vi "Joint Limits.vi"(8 "Side":T1, 11 "Joints":dbl[](array[numeric]) format="%.3f") -> (0 "In Range":bool)   [LabVIEW 2013]
uses:
  ROS/Code/SubVIs/BaxterSide.ctl
  Arm Globals.vi
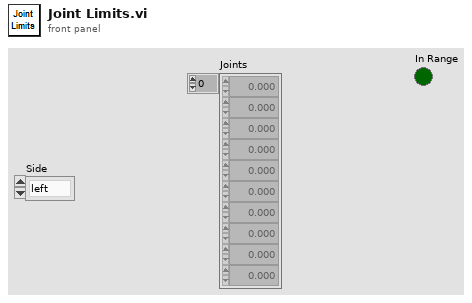
[diagram p1: front panel]
types:
  T1 = typedef "BaxterSide.ctl" = enum16{"left", "right"}
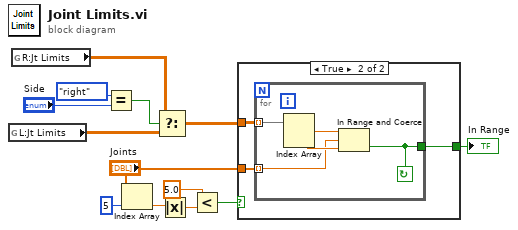
[diagram p0: block diagram]
diagram:
  n1 = global read "Arm Globals.vi" "L:Jt Limits"() -> (w1:dbl[][])
  n2 = global read "Arm Globals.vi" "R:Jt Limits"() -> (w6:dbl[][])
  n3 = Equal?(x=BaxterSide."right", y="Side") -> (x = y?=w4:bool)
  n4 = Index Array(array="Joints", index=5) -> (element=w10:dbl)
  n5 = Select(t=w6, s=w4, f=w1) -> (s? t:f=w5:dbl[][])
  n6 = Absolute Value(x=w10) -> (abs(x)=w9:dbl)
  n7 = Less?(x=5.0, y=w9) -> (x < y?=w7:bool)
  n8 = case shown="True" w7 {
    selector: w7 -> [w14 _]
    tunnel: "Joints" -> [_ w17]
    tunnel: w5 -> [_ w16]
    tunnel: [w14 w15] -> w13
    frame False {
      # "Singularity check\nat joint W1"
    }
    frame True {
      n9 = for {
        tunnel: w16 -> [w22] mode=indexing
        tunnel: w17 -> [w19] mode=indexing
        tunnel: [w18] -> w15
        stop <- w18 continue-if-true
        n10 = Index Array(array=w22) -> (element #1=w21:dbl, element #2=w20:dbl)  [unwired: 2 in]
        n11 = In Range and Coerce(upper limit=w21, x=w19, lower limit=w20) -> (In Range?=w18:bool)  [unwired: 1 out]
      }
    }
  }
  "In Range" <- w13
